vi "Test Assert Equal Value (Typedef).vi"(8 "error in":errorcluster) -> (0 "error out":errorcluster)   [LabVIEW 2009]
uses:
  <vilib>/Utility/error.llb/ErrWarn.ctl
  <vilib>/Utility/error.llb/DialogTypeEnum.ctl
  <vilib>/picture/picture.llb/imagedata.ctl
  <vilib>/Utility/miscctls.llb/LVBoundsTypeDef.ctl
  classes/Assert/Assert Equal Value_Variant.vi
  classes/Assert/Assert.lvclass
  classes/Test/Test.lvclass
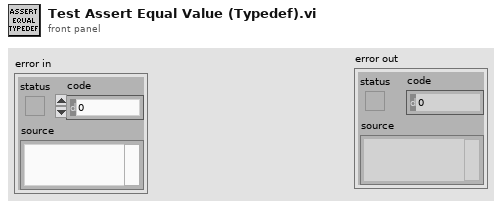
[diagram p1: front panel]
types:
  T1 = typedef "LVBoundsTypeDef.ctl" = cluster{"Width":u32, "Height":u32}
  T2 = cluster{"image type":i32, "image depth":i32, "image":u8[], "mask":u8[], "colors":u32[], "Rectangle":cluster{"left":i16, "top":i16, "right":i16, "bottom":i16}}
  T3 = typedef "imagedata.ctl" = cluster{"image type":i32, "image depth":i32, "image":u8[], "mask":u8[], "colors":u32[], "Rectangle":cluster{"left":i16, "top":i16, "right":i16, "bottom":i16}}
  T4 = enum16{"no dialog", "OK message", "continue or stop message", "auto error handling dialog", "OK message + warnings", "continue/stop + warnings"}
  T5 = typedef "DialogTypeEnum.ctl" = enum16{"no dialog", "OK message", "continue or stop message", "auto error handling dialog", "OK message + warnings", "continue/stop + warnings"}
  T6 = typedef "ErrWarn.ctl" = bool
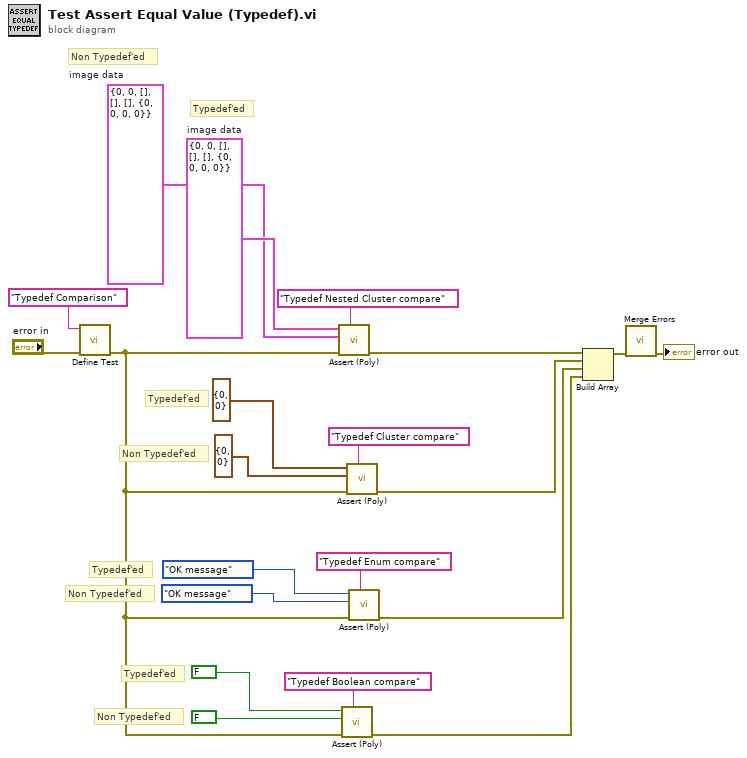
[diagram p0: block diagram]
diagram:
  w8 = T2 {"image type"=0, "image depth"=0, "image"=[], "mask"=[], "colors"=[], "Rectangle"={"left"=0, "top"=0, "right"=0, "bottom"=0}}  # image data
  w9 = T3 {"image type"=0, "image depth"=0, "image"=[], "mask"=[], "colors"=[], "Rectangle"={"left"=0, "top"=0, "right"=0, "bottom"=0}}  # image data
  # "Non Typedef'ed"
  # "Typedef'ed"
  # "Non Typedef'ed"
  # "Typedef'ed"
  # "Non Typedef'ed"
  # "Typedef'ed"
  # "Non Typedef'ed"
  # "Typedef'ed"
  n1 = call "Define Test.vi"("error in (no error)"="error in", "Label (VI Title)"="Typedef Comparison" ("Label")) -> ("error out"=w6:errorcluster)  [unwired: 9 in]
  n2 = call-poly "Assert (Poly).vi"("Label"="Typedef Nested Cluster compare", "error in (no error)"=w6, "Y"=w8, "X"=w9) -> ("error out"=w18:errorcluster)  [unwired: 7 in]
  n3 = call-poly "Assert (Poly).vi"("Label"="Typedef Boolean compare", "error in (no error)"=w6, "Y"=FALSE ("Boolean"), "X"=T6 FALSE ("Boolean")) -> ("error out"=w12:errorcluster)  [unwired: 7 in]
  n4 = call-poly "Assert (Poly).vi"("Label"="Typedef Cluster compare", "error in (no error)"=w6, "Y"=cluster{"Width":u32, "Height":u32} {"Width"=0, "Height"=0} ("Bounds"), "X"=T1 {"Width"=0, "Height"=0} ("Bounds")) -> ("error out"=w5:errorcluster)  [unwired: 7 in]
  n5 = call-poly "Assert (Poly).vi"("Label"="Typedef Enum compare", "error in (no error)"=w6, "Y"=T4."OK message" ("type of dialog (OK msg:1)"), "X"=DialogTypeEnum."OK message" ("type of dialog (OK msg:1)")) -> ("error out"=w17:errorcluster)  [unwired: 7 in]
  n6 = Build Array(w18, w5, w17, w12) -> (w2:errorcluster[])
  n7 = call <vilib>:"Merge Errors.vi"("error array in"=w2) -> ("error out"=→"error out":errorcluster)  [unwired: 6 in]
